vi "Sort Record Entries.vi"(4 "Entries":string[](array[string])) -> (1 "Sorted Entries":string[](array[string]))   [LabVIEW 2013, in "Data Log Fetcher.lvlib"]
uses:
  Data Log Fetcher.lvlib
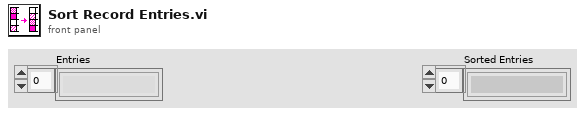
[diagram p1: front panel]
types:
  T1 = enum16{"JAN", "FEB", "MAR", "APR", "MAY", "JUN", "JUL", "AUG", "SEP", "OCT", "NOV", "DEC"}
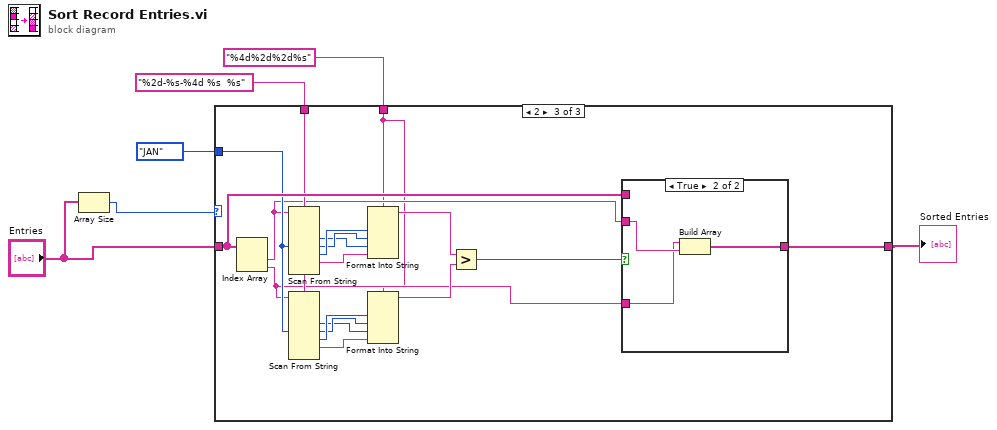
[diagram p0: block diagram]
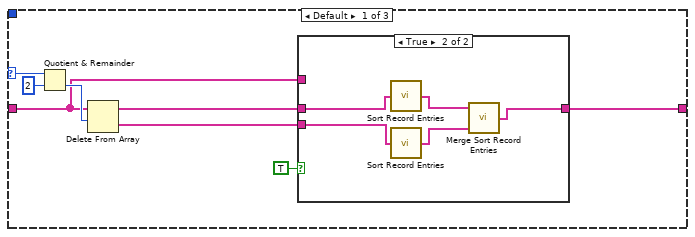
[diagram p2: hidden frame]
diagram:
  n1 = Array Size(array="Entries") -> (size(s)=w4:i32)
  n2 = case shown="2" w4 {
    selector: w4 -> [w14 _ _]
    tunnel: "Entries" -> [w7 w21 w38]
    tunnel: [w12 w21 w39] -> w5
    tunnel: "%2d-%s-%4d %s  %s" ("format string") -> [_ _ w37]
    tunnel: T1."JAN" ("Months") -> [_ _ w36]
    tunnel: "%4d%2d%2d%s" ("format string") -> [_ _ w22]
    frame Default {
      n3 = Quotient & Remainder(x=w14, y=2) -> (floor(x/y)=w11:i32)  [unwired: 1 out]
      n4 = Delete From Array(array=w7, length=w11) -> (deleted portion=w9:string[], array with subset deleted=w10:string[])  [unwired: 1 in]
      n5 = case shown="True" TRUE {
        tunnel: [w15 w20] -> w12
        tunnel: w10 -> [_ w19]
        tunnel: w9 -> [_ w18]
        tunnel: w7 -> [w15 _]
        frame False {
        }
        frame True {
          n6 = call "Sort Record Entries.vi"("Entries"=w19) -> ("Sorted Entries"=w17:string[])  [unwired: 4 in]
          n7 = call "Sort Record Entries.vi"("Entries"=w18) -> ("Sorted Entries"=w16:string[])  [unwired: 4 in]
          n8 = call "Merge Sort Record Entries.vi"("Sorted Entries A"=w17, "Sorted Entries B"=w16) -> ("Sorted Entries"=w20:string[])  [unwired: 5 in]
        }
      }
    }
    frame 1 {
    }
    frame 2 {
      n9 = Index Array(array=w38) -> (element #1=w24:string, element #2=w23:string)  [unwired: 2 in]
      n10 = Scan From String(format string=w37, input string=w24, default 2=w36) -> (output 1=w33:i32, output 2=w34:T1, output 3=w35:i32, output 4=w32:string)  [unwired: 7 in, 3 out]
      n11 = Scan From String(format string=w37, input string=w23, default 2=w36) -> (output 1=w29:i32, output 2=w30:T1, output 3=w31:i32, output 4=w28:string)  [unwired: 7 in, 3 out]
      n12 = Format Into String(format string=w22, w35, w34, w33, w32) -> (resulting string=w27:string)  [unwired: 2 in, 1 out]
      n13 = Format Into String(format string=w22, w31, w30, w29, w28) -> (resulting string=w26:string)  [unwired: 2 in, 1 out]
      n14 = Greater?(x=w27, y=w26) -> (0:w25:bool)
      n15 = case shown="True" w25 {
        tunnel: [w40 w43] -> w39
        tunnel: w24 -> [_ w42]
        tunnel: w23 -> [_ w41]
        tunnel: w38 -> [w40 _]
        frame False {
        }
        frame True {
          n16 = Build Array(w41, w42) -> (w43:string[])
        }
      }
    }
  }
  "Sorted Entries" <- w5
